vi "subvi 7seg.vi"(0 "Numeric Control":i32) -> (1 "left bottom":bool, 2 "top":bool, 3 "left top":bool, 4 "point":bool, 5 "right top":bool, 6 "middle":bool, 7 "right bottom":bool, 8 "bottom":bool)   [LabVIEW 2015]
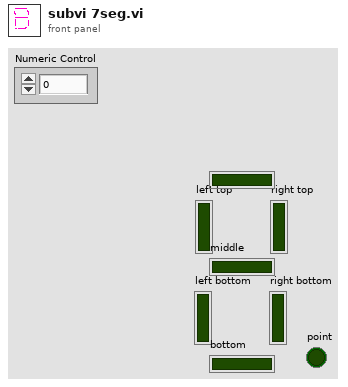
[diagram p1: front panel]
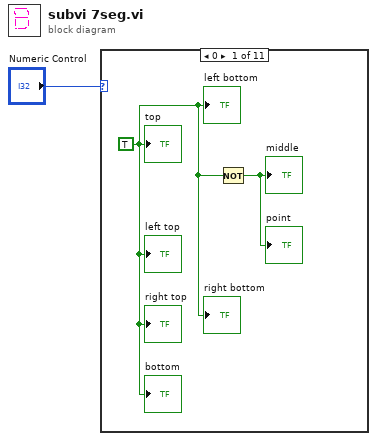
[diagram p0: block diagram]
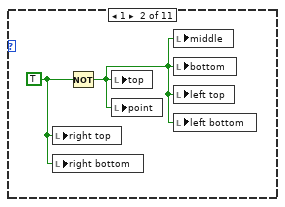
[diagram p2: hidden frame]
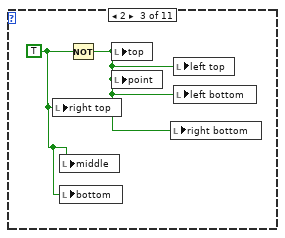
[diagram p3: hidden frame]
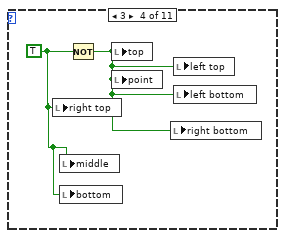
[diagram p4: hidden frame]
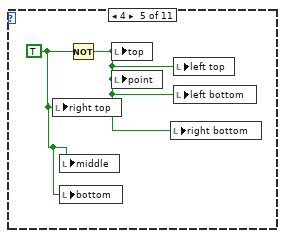
[diagram p5: hidden frame]
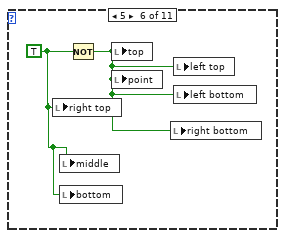
[diagram p6: hidden frame]
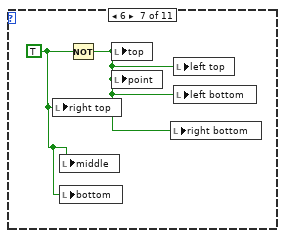
[diagram p7: hidden frame]
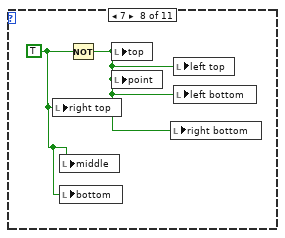
[diagram p8: hidden frame]
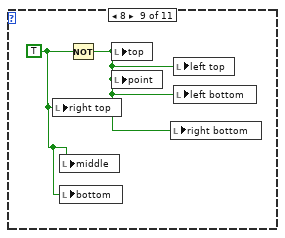
[diagram p9: hidden frame]
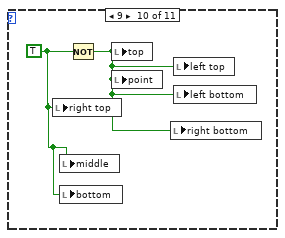
[diagram p10: hidden frame]
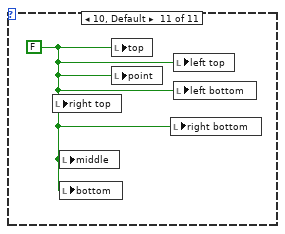
[diagram p11: hidden frame]
diagram:
  n1 = case shown="0" "Numeric Control" {
    frame 0 {
      w2 = TRUE
      n2 = Not(x=w2) -> (.not. x?=→"middle" →"point":bool)
      "bottom" <- w2
      "top" <- w2
      "left top" <- w2
      "right top" <- w2
      "left bottom" <- w2
      "right bottom" <- w2
    }
    frame 1 {
      w5 = TRUE
      n3 = local write "right top"(w5) -> ()
      n4 = local write "right bottom"(w5) -> ()
      n5 = Not(x=w5) -> (.not. x?=w4:bool)
      n6 = local write "top"(w4) -> ()
      n7 = local write "point"(w4) -> ()
      n8 = local write "middle"(w4) -> ()
      n9 = local write "bottom"(w4) -> ()
      n10 = local write "left top"(w4) -> ()
      n11 = local write "left bottom"(w4) -> ()
    }
    frame 2 {
      w7 = TRUE
      n12 = local write "right top"(w7) -> ()
      n13 = local write "middle"(w7) -> ()
      n14 = local write "bottom"(w7) -> ()
      n15 = Not(x=w7) -> (.not. x?=w6:bool)
      n16 = local write "top"(w6) -> ()
      n17 = local write "point"(w6) -> ()
      n18 = local write "right bottom"(w6) -> ()
      n19 = local write "left top"(w6) -> ()
      n20 = local write "left bottom"(w6) -> ()
    }
    frame 3 {
      w9 = TRUE
      n21 = local write "right top"(w9) -> ()
      n22 = local write "middle"(w9) -> ()
      n23 = local write "bottom"(w9) -> ()
      n24 = Not(x=w9) -> (.not. x?=w8:bool)
      n25 = local write "top"(w8) -> ()
      n26 = local write "point"(w8) -> ()
      n27 = local write "right bottom"(w8) -> ()
      n28 = local write "left top"(w8) -> ()
      n29 = local write "left bottom"(w8) -> ()
    }
    frame 4 {
      w11 = TRUE
      n30 = local write "right top"(w11) -> ()
      n31 = local write "middle"(w11) -> ()
      n32 = local write "bottom"(w11) -> ()
      n33 = Not(x=w11) -> (.not. x?=w10:bool)
      n34 = local write "top"(w10) -> ()
      n35 = local write "point"(w10) -> ()
      n36 = local write "right bottom"(w10) -> ()
      n37 = local write "left top"(w10) -> ()
      n38 = local write "left bottom"(w10) -> ()
    }
    frame 5 {
      w13 = TRUE
      n39 = local write "right top"(w13) -> ()
      n40 = local write "middle"(w13) -> ()
      n41 = local write "bottom"(w13) -> ()
      n42 = Not(x=w13) -> (.not. x?=w12:bool)
      n43 = local write "top"(w12) -> ()
      n44 = local write "point"(w12) -> ()
      n45 = local write "right bottom"(w12) -> ()
      n46 = local write "left top"(w12) -> ()
      n47 = local write "left bottom"(w12) -> ()
    }
    frame 6 {
      w15 = TRUE
      n48 = local write "right top"(w15) -> ()
      n49 = local write "middle"(w15) -> ()
      n50 = local write "bottom"(w15) -> ()
      n51 = Not(x=w15) -> (.not. x?=w14:bool)
      n52 = local write "top"(w14) -> ()
      n53 = local write "point"(w14) -> ()
      n54 = local write "right bottom"(w14) -> ()
      n55 = local write "left top"(w14) -> ()
      n56 = local write "left bottom"(w14) -> ()
    }
    frame 7 {
      w17 = TRUE
      n57 = local write "right top"(w17) -> ()
      n58 = local write "middle"(w17) -> ()
      n59 = local write "bottom"(w17) -> ()
      n60 = Not(x=w17) -> (.not. x?=w16:bool)
      n61 = local write "top"(w16) -> ()
      n62 = local write "point"(w16) -> ()
      n63 = local write "right bottom"(w16) -> ()
      n64 = local write "left top"(w16) -> ()
      n65 = local write "left bottom"(w16) -> ()
    }
    frame 8 {
      w19 = TRUE
      n66 = local write "right top"(w19) -> ()
      n67 = local write "middle"(w19) -> ()
      n68 = local write "bottom"(w19) -> ()
      n69 = Not(x=w19) -> (.not. x?=w18:bool)
      n70 = local write "top"(w18) -> ()
      n71 = local write "point"(w18) -> ()
      n72 = local write "right bottom"(w18) -> ()
      n73 = local write "left top"(w18) -> ()
      n74 = local write "left bottom"(w18) -> ()
    }
    frame 9 {
      w21 = TRUE
      n75 = local write "right top"(w21) -> ()
      n76 = local write "middle"(w21) -> ()
      n77 = local write "bottom"(w21) -> ()
      n78 = Not(x=w21) -> (.not. x?=w20:bool)
      n79 = local write "top"(w20) -> ()
      n80 = local write "point"(w20) -> ()
      n81 = local write "right bottom"(w20) -> ()
      n82 = local write "left top"(w20) -> ()
      n83 = local write "left bottom"(w20) -> ()
    }
    frame 10, Default {
      w22 = FALSE
      n84 = local write "right top"(w22) -> ()
      n85 = local write "middle"(w22) -> ()
      n86 = local write "bottom"(w22) -> ()
      n87 = local write "top"(w22) -> ()
      n88 = local write "point"(w22) -> ()
      n89 = local write "right bottom"(w22) -> ()
      n90 = local write "left top"(w22) -> ()
      n91 = local write "left bottom"(w22) -> ()
    }
  }
